vi "Clusters.vi"() -> ()   [LabVIEW 2011]
uses:
  LV JSON.lvlib
panel:
  out "Array of clusters out":T1(array[cluster])
  out "Array of clusters OK?":bool
  out "NestedCluster OK?":bool
  out "NestedCluster out":T2 {"Slide" format="%#_9g"}
  out "NestedCluster JSON":string
  in  "NestedCluster":T2={"Slide"=5.6566, "Simple Cluster"={"Numeric"=352.0, "Boolean"=TRUE, "enum2"=enum."second", "Path"=path "C:/test", "String"="\"example string\"\npart 2"}} {"Slide" step=0.0001 scale=0.0..10.0}
  out "Simple Cluster OK?":bool
  out "Simple Cluster out":T3
  out "JSON Simple Cluster":string
  in  "Simple Cluster":T3={"Numeric"=251.0, "Boolean"=TRUE, "Enum"=enum."second", "Path"=path "C:/test", "String"="example string", "DBLarray"=[1.0, 2.0, 3.0], "Comments"="asdfsa\nasdf\n"}
  out "Cluster 2 OK?":bool
  out "Cluster 2":T4
  in  "Cluster 2":T4={"abc"={"def"=1.0, "ghi"=2.0}, "jkl"=3.0}
  out "Cluster 2 JSON":string
  out "DBLArray OK?":bool
  out "DBLArray Out":dbl[](array[numeric])
  out "DBLArray JSON":string
  in  "DBLarray":dbl[](array[numeric])=[1.0, 2.0, 3.0]
  out "Cluster of Arrays OK?":bool
  out "Cluster of Arrays out":cluster{"DBLarray":dbl[], "DBLarray 2":dbl[]}
  out "Cluster of Arrays JSON":string
  in  "Cluster of Arrays":cluster{"DBLarray":dbl[], "DBLarray 2":dbl[]}={"DBLarray"=[1.0, 2.0, 3.0], "DBLarray 2"=[2.0, 4.0, 6.0]}
  out "Path OK?":bool
  out "Path Out":path
  out "Path JSON":string
  in  "Path":path=path "D:/\"My Data\"/test"
  out "Array of clusters (JSON)":string
  in  "Array of clusters":T1(array[cluster])=[{"Numeric"=51.0, "Boolean"=FALSE, "Enum"=enum."second", "Path"=path "C:/t est", "String"="examplestring"}, {"Numeric"=121.0, "Boolean"=TRUE, "Enum"=enum."second", "Path"=path "D:/stest", "String"="asdfasd"}]
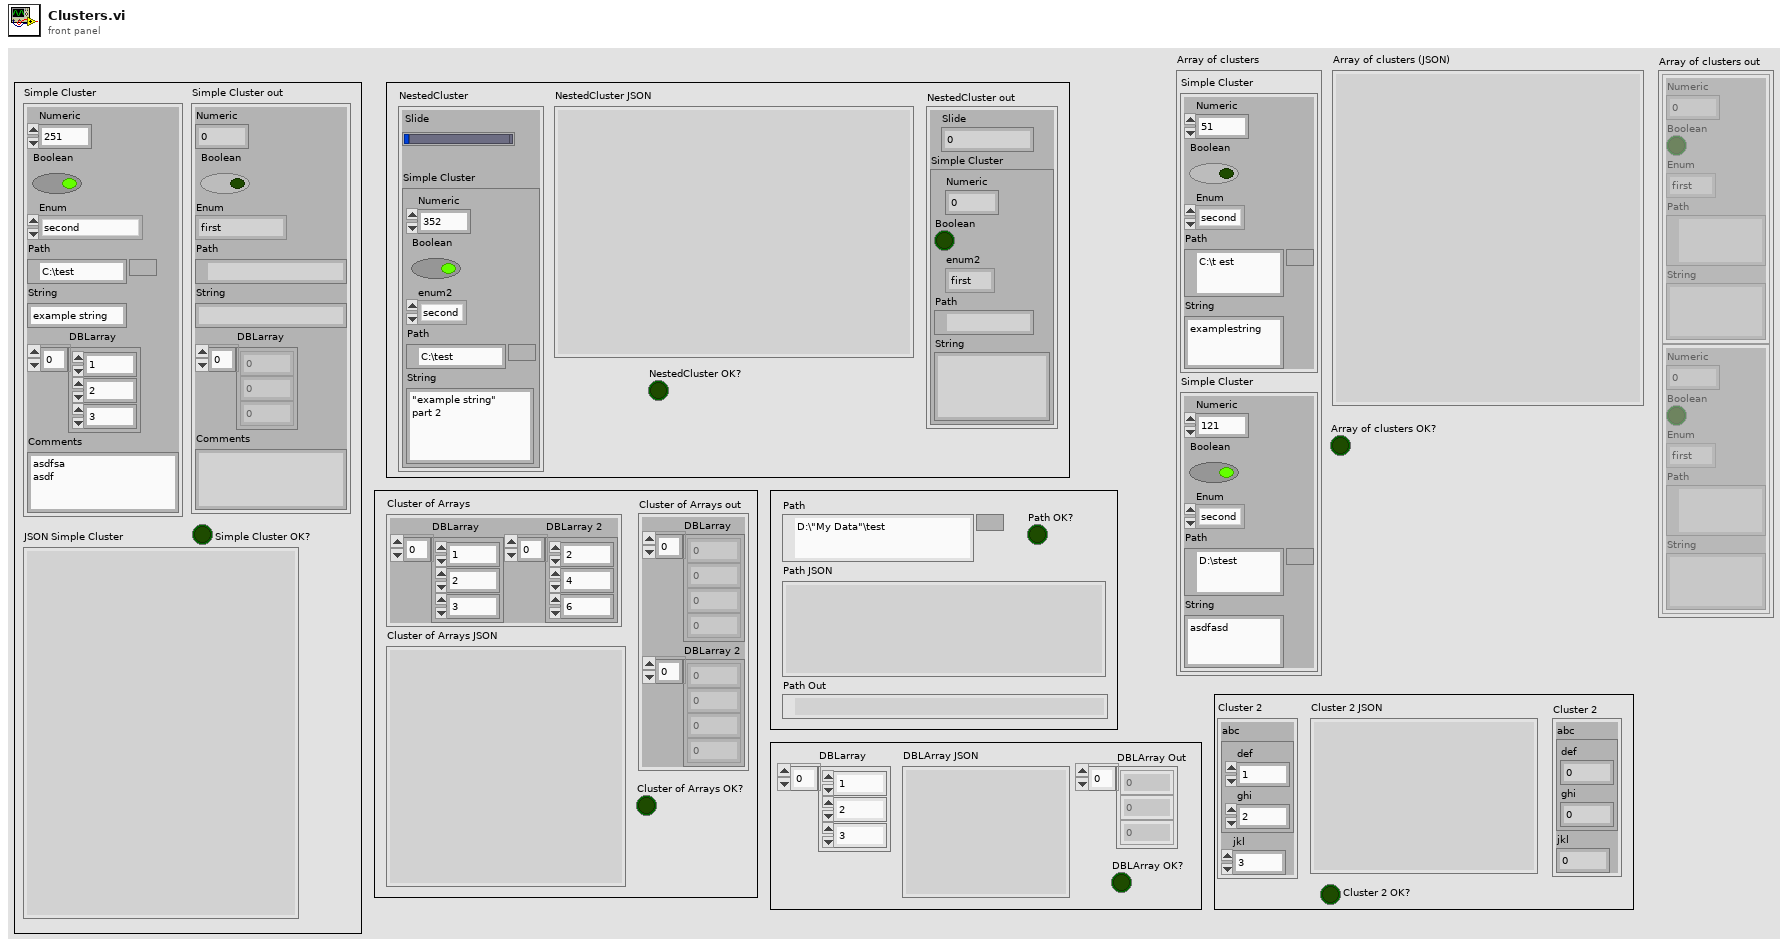
[diagram p1: front panel]
types:
  T1 = cluster{"Numeric":dbl, "Boolean":bool, "Enum":enum16{"first", "second"}, "Path":path, "String":string}[]
  T2 = cluster{"Slide":dbl, "Simple Cluster":cluster{"Numeric":dbl, "Boolean":bool, "enum2":enum16{"first", "second"}, "Path":path, "String":string}}
  T3 = cluster{"Numeric":dbl, "Boolean":bool, "Enum":enum16{"first", "second"}, "Path":path, "String":string, "DBLarray":dbl[], "Comments":string}
  T4 = cluster{"abc":cluster{"def":dbl, "ghi":dbl}, "jkl":dbl}
  T5 = cluster{"Slide":bool, "Simple Cluster":cluster{"Numeric":bool, "Boolean":bool, "enum2":bool, "Path":bool, "String":bool}}
  T6 = cluster{"abc":cluster{"def":bool, "ghi":bool}, "jkl":bool}
  T7 = cluster{"Numeric":bool, "Boolean":bool, "Enum":bool, "Path":bool, "String":bool}[]
  T8 = cluster{"Numeric":bool, "Boolean":bool, "Enum":bool, "Path":bool, "String":bool, "DBLarray":bool[], "Comments":bool}
  T9 = cluster{"Numeric":bool, "Boolean":bool, "enum2":bool, "Path":bool, "String":bool}
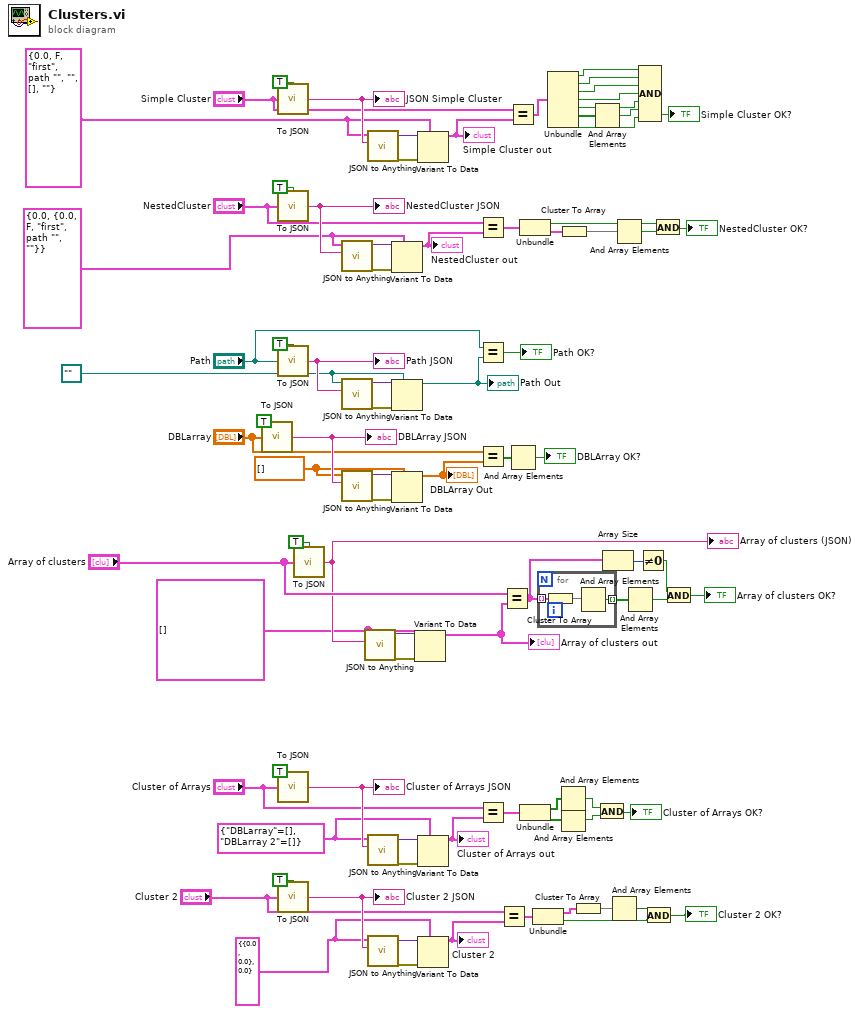
[diagram p0: block diagram]
diagram:
  w1 = T4 {"abc"={"def"=0.0, "ghi"=0.0}, "jkl"=0.0} ("Cluster 2")
  w4 = T1 [] ("Array of clusters")
  w5 = cluster{"DBLarray":dbl[], "DBLarray 2":dbl[]} {"DBLarray"=[], "DBLarray 2"=[]} ("Cluster of Arrays")
  w10 = dbl[] [] ("DBLarray")
  w11 = path "" ("Path")
  w12 = T2 {"Slide"=0.0, "Simple Cluster"={"Numeric"=0.0, "Boolean"=FALSE, "enum2"=enum."first", "Path"=path "", "String"=""}} ("NestedCluster")
  w13 = T3 {"Numeric"=0.0, "Boolean"=FALSE, "Enum"=enum."first", "Path"=path "", "String"="", "DBLarray"=[], "Comments"=""} ("Simple Cluster")
  n1 = call "To JSON.vi"("Anything"="DBLarray", "Pretty Print (F)"=TRUE) -> ("JSON"=w67:string)
  "DBLArray JSON" <- w67
  n2 = call "To JSON.vi"("Anything"="Simple Cluster", "Pretty Print (F)"=TRUE) -> ("JSON"=w69:string)
  "JSON Simple Cluster" <- w69
  n3 = call "To JSON.vi"("Anything"="NestedCluster", "Pretty Print (F)"=TRUE) -> ("JSON"=w63:string)
  "NestedCluster JSON" <- w63
  n4 = call "To JSON.vi"("Anything"="Path", "Pretty Print (F)"=TRUE) -> ("JSON"=w68:string)
  "Path JSON" <- w68
  n5 = call "To JSON.vi"("Anything"="Cluster of Arrays", "Pretty Print (F)"=TRUE) -> ("JSON"=w66:string)
  "Cluster of Arrays JSON" <- w66
  n6 = call "To JSON.vi"("Anything"="Cluster 2", "Pretty Print (F)"=TRUE) -> ("JSON"=w44:string)
  "Cluster 2 JSON" <- w44
  n7 = call "To JSON.vi"("Anything"="Array of clusters", "Pretty Print (F)"=TRUE) -> ("JSON"=w15:string)
  "Array of clusters (JSON)" <- w15
  n8 = call "JSON to Anything.vi"("JSON Object"=w63, "Type"=w12) -> ("error out"=w65:errorcluster, "Variant"=w64:variant)  [unwired: 6 in, 2 out]
  n9 = call "JSON to Anything.vi"("JSON Object"=w68, "Type"=w11) -> ("error out"=w81:errorcluster, "Variant"=w82:variant)  [unwired: 6 in, 2 out]
  n10 = call "JSON to Anything.vi"("JSON Object"=w67, "Type"=w10) -> ("error out"=w84:errorcluster, "Variant"=w83:variant)  [unwired: 6 in, 2 out]
  n11 = call "JSON to Anything.vi"("JSON Object"=w15, "Type"=w4) -> ("error out"=w2:errorcluster, "Variant"=w3:variant)  [unwired: 6 in, 2 out]
  n12 = call "JSON to Anything.vi"("JSON Object"=w69, "Type"=w13) -> ("error out"=w77:errorcluster, "Variant"=w78:variant)  [unwired: 6 in, 2 out]
  n13 = call "JSON to Anything.vi"("JSON Object"=w66, "Type"=w5) -> ("error out"=w79:errorcluster, "Variant"=w80:variant)  [unwired: 6 in, 2 out]
  n14 = call "JSON to Anything.vi"("JSON Object"=w44, "Type"=w1) -> ("error out"=w86:errorcluster, "Variant"=w85:variant)  [unwired: 6 in, 2 out]
  n15 = Variant To Data(error in=w65, type=w12, Variant=w64) -> (data=w23:T2)  [unwired: 1 out]
  "NestedCluster out" <- w23
  n16 = Variant To Data(error in=w81, type=w11, Variant=w82) -> (data=w61:path)  [unwired: 1 out]
  "Path Out" <- w61
  n17 = Variant To Data(error in=w84, type=w10, Variant=w83) -> (data=w51:dbl[])  [unwired: 1 out]
  "DBLArray Out" <- w51
  n18 = Variant To Data(error in=w2, type=w4, Variant=w3) -> (data=w17:T1)  [unwired: 1 out]
  "Array of clusters out" <- w17
  n19 = Variant To Data(error in=w77, type=w13, Variant=w78) -> (data=w36:T3)  [unwired: 1 out]
  "Simple Cluster out" <- w36
  n20 = Variant To Data(error in=w79, type=w5, Variant=w80) -> (data=w59:cluster{"DBLarray":dbl[], "DBLarray 2":dbl[]})  [unwired: 1 out]
  "Cluster of Arrays out" <- w59
  n21 = Variant To Data(error in=w86, type=w1, Variant=w85) -> (data=w45:T4)  [unwired: 1 out]
  "Cluster 2" <- w45
  n22 = Equal?(x="NestedCluster", y=w23) -> (x = y?=w24:T5)
  n23 = Equal?(x="Path", y=w61) -> (x = y?=→"Path OK?":bool)
  n24 = Equal?(x="DBLarray", y=w51) -> (x = y?=w49:bool[])
  n25 = Equal?(x="Cluster of Arrays", y=w59) -> (x = y?=w57:cluster{"DBLarray":bool[], "DBLarray 2":bool[]})
  n26 = Equal?(x="Cluster 2", y=w45) -> (x = y?=w46:T6)
  n27 = Equal?(x="Array of clusters", y=w17) -> (x = y?=w9:T7)
  n28 = Equal?(x="Simple Cluster", y=w36) -> (x = y?=w34:T8)
  n29 = And Array Elements(Boolean array=w49) -> (logical AND=→"DBLArray OK?":bool)
  n30 = Unbundle(w24) -> ("Slide"=w21:bool, "Simple Cluster"=w20:T9)
  n31 = Unbundle(w57) -> ("DBLarray"=w55:bool[], "DBLarray 2"=w56:bool[])
  n32 = Unbundle(w46) -> ("abc"=w41:cluster{"def":bool, "ghi":bool}, "jkl"=w42:bool)
  n33 = for {
    tunnel: w9 -> [w89] mode=indexing
    tunnel: [w88] -> w14 mode=indexing
    n34 = Cluster To Array(cluster=w89) -> (array=w87:bool[])
    n35 = And Array Elements(Boolean array=w87) -> (logical AND=w88:bool)
  }
  n36 = Unbundle(w34) -> ("Numeric"=w27:bool, "Boolean"=w28:bool, "Enum"=w29:bool, "Path"=w30:bool, "String"=w31:bool, "DBLarray"=w32:bool[], "Comments"=w33:bool)
  n37 = And Array Elements(Boolean array=w55) -> (logical AND=w54:bool)
  n38 = And Array Elements(Boolean array=w56) -> (logical AND=w53:bool)
  n39 = Cluster To Array(cluster=w20) -> (array=w19:bool[])
  n40 = Cluster To Array(cluster=w41) -> (array=w40:bool[])
  n41 = And Array Elements(Boolean array=w32) -> (logical AND=w37:bool)
  n42 = And(x=w54, y=w53) -> (x .and. y?=→"Cluster of Arrays OK?":bool)
  n43 = Array Size(array=w9) -> (size(s)=w7:i32)
  n44 = And Array Elements(Boolean array=w40) -> (logical AND=w47:bool)
  n45 = And Array Elements(Boolean array=w19) -> (logical AND=w25:bool)
  n46 = And Array Elements(Boolean array=w14) -> (logical AND=w18:bool)
  n47 = Not Equal To 0?(x=w7) -> (x != 0?=w6:bool)
  n48 = Compound Arithmetic op=AND(w27, w28, w29, w30, w31, w37, w33) -> (→"Simple Cluster OK?":bool)
  n49 = And(x=w47, y=w42) -> (x .and. y?=→"Cluster 2 OK?":bool)
  n50 = And(x=w21, y=w25) -> (x .and. y?=→"NestedCluster OK?":bool)
  n51 = And(x=w6, y=w18) -> (x .and. y?=→"Array of clusters OK?":bool)
